vi "Lego-Challenge-1.vi"   [LabVIEW 2014, in "Diaz_Razo_5th_LegoRobotics_11-29-16.lvrbt"]
uses:
  Diaz_Razo_5th_LegoRobotics_11-29-16.lvrbt
  <vilib>/NXT/Block Support/NXT_InputPort.ctl
  <vilib>/NXT/Block Support/NXT_OutputPort.ctl
  <vilib>/NXT/NXTIO Xnodes/NXTIONodeSubVIs/NXTMoveMotors.vi
  <vilib>/NXT/NXTIO Xnodes/NXTIONodeSubVIs/NXTStopMotors.vi
  <vilib>/NXT/Subs/LVHSConnector.ctl
  <vilib>/NXT/NXTIO Xnodes/AddressXNode/NXTIOAddress.xnode
  <vilib>/NXT/NXTIO Xnodes/NXTIOXNode/NXTIO.xnode
  <vilib>/NXT/LegoClasses/BrickReference/BrickReference.lvclass
types:
  T1 = typedef "NXT_OutputPort.ctl" = u8
  T2 = typedef "NXT_InputPort.ctl" = u32
  T3 = typedef "LVHSConnector.ctl" = refnum<class "BrickReference.lvclass">
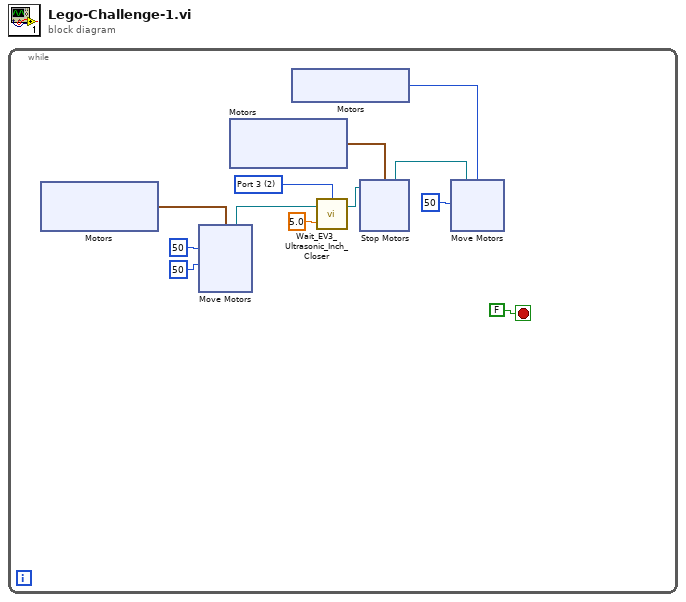
[diagram p0: block diagram]
diagram:
  n1 = while {
    stop <- FALSE stop-if-true
    w1 = T2 2 items=["Port 1", "Port 2", "Port 3", "Port 4"] ("Port (Port 1)")
    n2 = xnode "Motors"() -> ("Motor"=w12:cluster{"Port":T1, "Port":T1})
    n3 = xnode "Move Motors"("Power/Speed 2"=i8 50, "Power/Speed 1"=i8 50, "Motors"=w12) -> ("NXT/EV3"=w10:T3)  [unwired: 1 in]
    n4 = xnode "Motors"() -> ("Motor"=w3:cluster{"Port":T1, "Port":T1})
    n5 = xnode "Motors"() -> ("Motor"=w8:T1)
    n6 = call <vilib>:"Wait_EV3_Ultrasonic_Inch_Closer.vi"("Inches (5)"=sgl 5.0, "NXT/EV3"=w10, "Port (Port 1)"=w1) -> ("NXT/EV3"=w2:T3)  [unwired: 1 in]
    n7 = xnode "Stop Motors"("Motors"=w3, "NXT/EV3"=w2) -> ("NXT/EV3"=w9:T3)
    n8 = xnode "Move Motors"("Power/Speed 1"=i8 50, "Motors"=w8, "NXT/EV3"=w9) -> ()  [unwired: 1 out]
  }
